vi "HumanDashReadSlow.vi"(8 "error in (no error)":errorcluster) -> (0 "error out":errorcluster)   [LabVIEW 2023]
doc: "Human Network\n\nInput\n --Error in \n\nOutput\n --Error out"
uses:
  <vilib>/Rock Robotics/Network Tables/NT Read Number.vi
  HumanGlobal.vi
  <vilib>/Rock Robotics/Network Tables/NT Write Number.vi
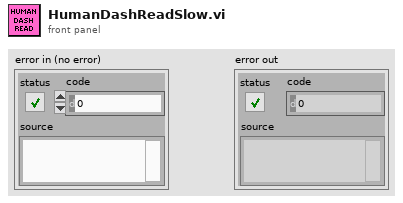
[diagram p1: front panel]
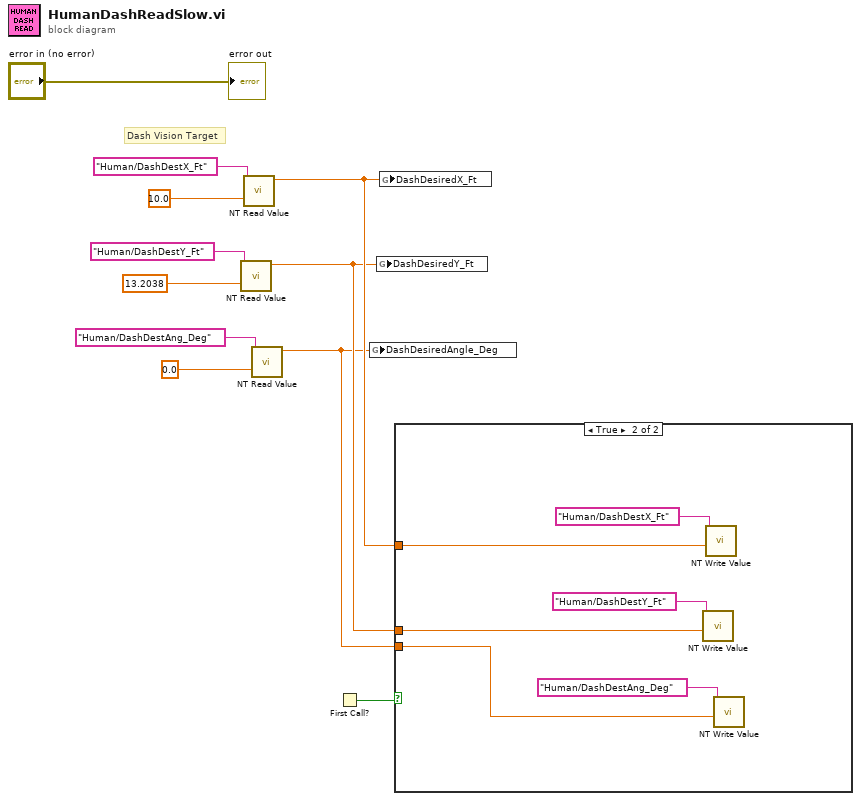
[diagram p0: block diagram]
diagram:
  # "Dash Vision Target"
  n1 = call-poly <vilib>:"NT Read Value.vi"("default value"=13.2038, "name"="Human/DashDestY_Ft") -> ("value"=w2:dbl)  [unwired: 7 in, 2 out]
  n2 = call-poly <vilib>:"NT Read Value.vi"("default value"=10.0, "name"="Human/DashDestX_Ft") -> ("value"=w3:dbl)  [unwired: 7 in, 2 out]
  n3 = call-poly <vilib>:"NT Read Value.vi"("default value"=0.0, "name"="Human/DashDestAng_Deg") -> ("value"=w1:dbl)  [unwired: 7 in, 2 out]
  n4 = First Call?() -> (First Call?: T/F=w4:bool)
  n5 = global write "HumanGlobal.vi" "DashDesiredAngle_Deg"(w1) -> ()
  n6 = global write "HumanGlobal.vi" "DashDesiredY_Ft"(w2) -> ()
  n7 = global write "HumanGlobal.vi" "DashDesiredX_Ft"(w3) -> ()
  n8 = case shown="True" w4 {
    tunnel: w3 -> [_ w14]
    tunnel: w2 -> [_ w13]
    tunnel: w1 -> [_ w12]
    frame False {
    }
    frame True {
      n9 = call-poly <vilib>:"NT Write Value.vi"("value"=w13, "name"="Human/DashDestY_Ft") -> ()  [unwired: 9 in, 1 out]
      n10 = call-poly <vilib>:"NT Write Value.vi"("value"=w14, "name"="Human/DashDestX_Ft") -> ()  [unwired: 9 in, 1 out]
      n11 = call-poly <vilib>:"NT Write Value.vi"("value"=w12, "name"="Human/DashDestAng_Deg") -> ()  [unwired: 9 in, 1 out]
    }
  }
  "error out" <- "error in (no error)"
